vi "MGI Running Average(SGL).vi"(5 "Averaging Size":i32, 6 "Average Type(FIR)":T1, 7 "Initialize? (F)":bool, 11 "Value":sgl) -> (3 "Average":sgl)   [LabVIEW 2020]
doc: "Keep a running average of the input value. Infinite Impulse Response requires less processing, but it takes infinite time to arrive at a steady state value. Finite Impulse Reponse maintains an array of the specified size but is able to output a mean.\nThis VI is a reentrant functional global.\n\nAuthored by Shawn Walpole\nsupport@mooregoodideas.com\nwww.mooregoodideas.com\n\nCopyright (c) 2010, Moore Good Ideas, Inc.\n\nAll rights reserved.\n\nRedistribution and use in source and binary forms, with or without modification, are permitted provided that the following conditions are met:\n\n * Redistributions of source code must retain the above copyright notice, this list of conditions and the following disclaimer.\n * Redistributions in binary form must reproduce the above copyright notice, this list of conditions and the following disclaimer in the documentation and/or other materials provided with the distribution.\n * Neither the name of Moore Good Ideas, Inc. nor the names of its contributors may be used to endorse or promote products derived from this software without specific prior written permission.\n\nTHIS SOFTWARE IS PROVIDED BY THE COPYRIGHT HOLDERS AND CONTRIBUTORS \"AS IS\" AND ANY EXPRESS OR IMPLIED WARRANTIES, INCLUDING, BUT NOT LIMITED TO, THE IMPLIED WARRANTIES OF MERCHANTABILITY AND FITNESS FOR A PARTICULAR PURPOSE ARE DISCLAIMED. IN NO EVENT SHALL THE COPYRIGHT OWNER OR CONTRIBUTORS BE LIABLE FOR ANY DIRECT, INDIRECT, INCIDENTAL, SPECIAL, EXEMPLARY, OR CONSEQUENTIAL DAMAGES (INCLUDING, BUT NOT LIMITED TO, PROCUREMENT OF SUBSTITUTE GOODS OR SERVICES; LOSS OF USE, DATA, OR PROFITS; OR BUSINESS INTERRUPTION) HOWEVER CAUSED AND ON ANY THEORY OF LIABILITY, WHETHER IN CONTRACT, STRICT LIABILITY, OR TORT (INCLUDING NEGLIGENCE OR OTHERWISE) ARISING IN ANY WAY OUT OF THE USE OF THIS SOFTWARE, EVEN IF ADVISED OF THE POSSIBILITY OF SUCH DAMAGE."
uses:
  <userlib>/_MGI/1D Array/MGI Average Type Enum.ctl
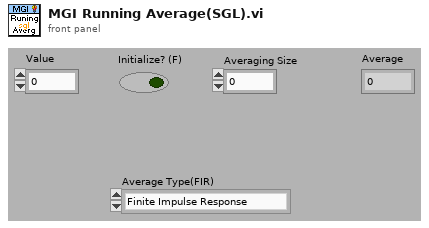
[diagram p1: front panel]
types:
  T1 = typedef "MGI Average Type Enum.ctl" = enum16{"Finite Impulse Response", "Infinite Impulse Response"}
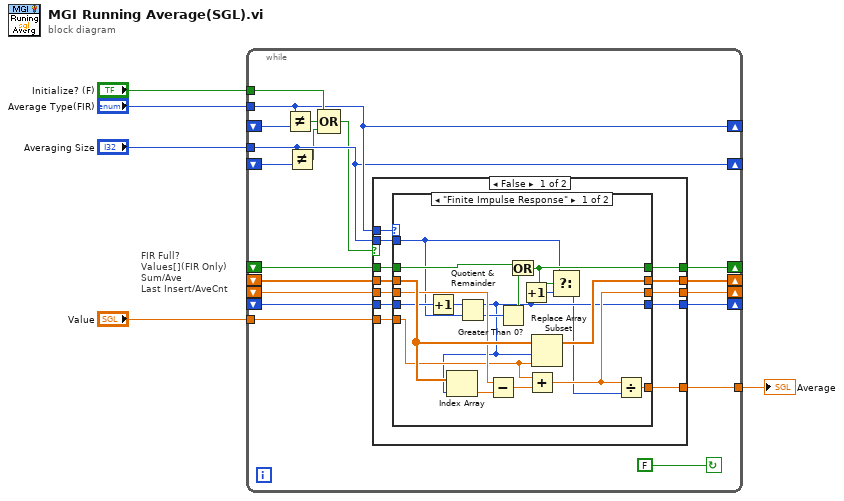
[diagram p0: block diagram]
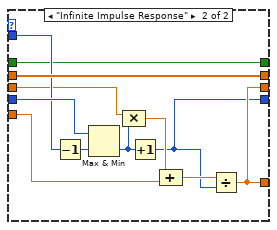
[diagram p2: hidden frame]
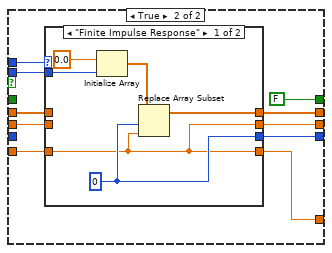
[diagram p3: hidden frame]
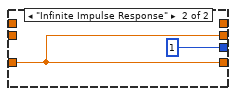
[diagram p4: hidden frame]
diagram:
  # "FIR Full?\nValues[](FIR Only)\nSum/Ave\nLast Insert/AveCnt"
  n1 = while {
    tunnel: "Averaging Size" -> [w12]
    tunnel: "Value" -> [w14]
    shift-left: _ -> [w17]
    shift-right: [w19] -> _
    tunnel: "Initialize? (F)" -> [w22]
    shift-left: _ -> [w8]
    shift-right: [w16] -> _
    tunnel: "Average Type(FIR)" -> [w13]
    shift-right: [w13] -> _
    shift-left: _ -> [w23]
    shift-right: [w20] -> _
    shift-left: _ -> [w18]
    shift-right: [w12] -> _
    shift-left: _ -> [w21]
    tunnel: [w15] -> w1
    shift-right: [w7] -> _
    shift-left: _ -> [w6]
    stop <- FALSE continue-if-true
    n2 = Not Equal?(x=w13, y=w23) -> (x != y?=w11:bool)
    n3 = Not Equal?(x=w12, y=w21) -> (x != y?=w9:bool)
    n4 = Compound Arithmetic op=OR(w22, w11, w9) -> (w10:bool)
    n5 = case shown="False" w10 {
      tunnel: [w30 w68] -> w20
      tunnel: w14 -> [w32 w71]
      tunnel: [w28 w70] -> w19
      tunnel: w18 -> [w35 _]
      tunnel: w17 -> [w34 w74]
      tunnel: w8 -> [w33 w72]
      tunnel: w12 -> [w31 w75]
      tunnel: w13 -> [w36 w76]
      tunnel: [w29 w73] -> w16
      tunnel: [w27 w69] -> w15
      tunnel: [w26 FALSE] -> w7
      tunnel: w6 -> [w25 _]
      frame False {
        n6 = case shown="\"Finite Impulse Response\"" w36 {
          tunnel: w35 -> [w52 w65]
          tunnel: w34 -> [w51 w62]
          tunnel: w33 -> [w53 w66]
          tunnel: w32 -> [w47 w61]
          tunnel: w31 -> [w40 w64]
          tunnel: [w39 w55] -> w30
          tunnel: [w49 w66] -> w29
          tunnel: [w46 w58] -> w28
          tunnel: [w45 w58] -> w27
          tunnel: [w41 w56] -> w26
          tunnel: w25 -> [w43 w56]
          frame "Finite Impulse Response" {
            n7 = Increment(x=w52) -> (x+1=w54:i32)
            n8 = Quotient & Remainder(x=w54, y=w40) -> (x-y*floor(x/y)=w39:i32, floor(x/y)=w44:i32)
            n9 = Index Array(array=w53, index=w39) -> (element=w50:sgl)
            n10 = Subtract(x=w51, y=w50) -> (x-y=w48:sgl)
            n11 = Greater Than 0?(x=w44) -> (x > 0?=w42:bool)
            n12 = Or(x=w43, y=w42) -> (x .or. y?=w41:bool)
            n13 = Increment(x=w39) -> (x+1=w37:i32)
            n14 = Add(x=w47, y=w48) -> (x+y=w46:sgl)
            n15 = Replace Array Subset(array=w53, new element=w47, index=w39) -> (w49:sgl[])
            n16 = Select(t=w40, s=w41, f=w37) -> (s? t:f=w38:i32)
            n17 = Divide(x=w46, y=w38) -> (x/y=w45:sgl)
          }
          frame "Infinite Impulse Response" {
            n18 = Decrement(x=w64) -> (x-1=w63:i32)
            n19 = Max & Min(x=w65, y=w63) -> (min(x,y)=w57:i32)  [unwired: 1 out]
            n20 = Compound Arithmetic op=MULTIPLY(w62, w57) -> (w60:sgl)
            n21 = Increment(x=w57) -> (x+1=w55:i32)
            n22 = Compound Arithmetic op=ADD(w60, w61) -> (w59:sgl)
            n23 = Divide(x=w59, y=w55) -> (x/y=w58:sgl)
          }
        }
      }
      frame True {
        n24 = case shown="\"Finite Impulse Response\"" w76 {
          tunnel: w75 -> [w82 _]
          tunnel: w74 -> [_ _]
          tunnel: [w79 _] -> w73
          tunnel: w72 -> [_ _]
          tunnel: w71 -> [w77 w84]
          tunnel: [w77 w84] -> w70
          tunnel: [w77 w84] -> w69
          tunnel: [w78 1] -> w68
          frame "Finite Impulse Response" {
            w78 = 0
            n25 = Initialize Array(sgl 0.0 ("Value"), w82) -> (w80:sgl[])
            n26 = Replace Array Subset(array=w80, new element=w77, index=w78) -> (w79:sgl[])
          }
          frame "Infinite Impulse Response" {
          }
        }
      }
    }
  }
  "Average" <- w1
